vi "SystemDefinitionSelectionDialog.vi"(8 "error in (no error)":errorcluster) -> (0 "error out":errorcluster, 2 "cancelled":bool, 3 "selected path":path)   [LabVIEW 2013, in "Simple Sequence Tools - Editor.lvlib"]
uses:
  Simple Sequence Tools - Editor.lvlib
  NationalInstruments.VeriStand.Internal
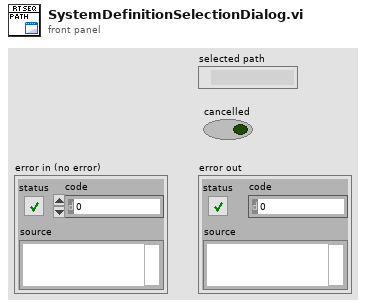
[diagram p1: front panel]
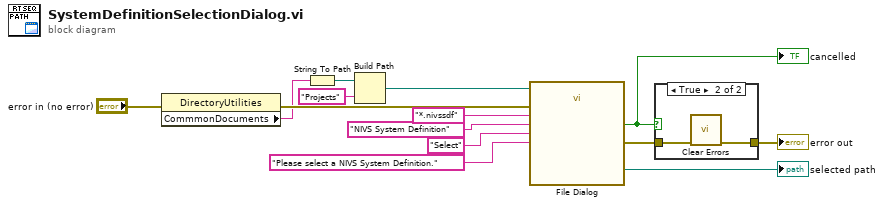
[diagram p0: block diagram]
diagram:
  n1 = property class="DirectoryUtilities"(error in="error in (no error)") -> (error out=w13:errorcluster, "CommmonDocuments"=w5:string)  [unwired: 1 in, 1 out]
  n2 = String To Path(string=w5) -> (path=w6:path)
  n3 = Build Path(base path=w6, name or relative path="Projects") -> (appended path=w8:path)
  n4 = call "File Dialog"("start path"=w8, "prompt"="Please select a NIVS System Definition.", "button label"="Select", "error in"=w13, "pattern (all files)"="*.nivssdf", "pattern label"="NIVS System Definition") -> ("selected path"=→"selected path":path, "cancelled"=w2:bool, "error out"=w3:errorcluster)  [unwired: 6 in, 1 out]
  "cancelled" <- w2
  n5 = case shown="True" w2 {
    tunnel: w3 -> [w15 w17]
    tunnel: [w15 w16] -> w1
    frame False {
    }
    frame True {
      n6 = call <vilib>:"Clear Errors.vi"("error in (no error)"=w17) -> ("error out"=w16:errorcluster)  [unwired: 6 in]
    }
  }
  "error out" <- w1
